vi "MEMR-Plot Gain Spectra.vi"(0 "Gain spectra in":cluster{"Freq (Hz)":dbl[], "Mag":dbl[][]}[](array[cluster]), 1 "Spectrum":refnum<vi>, 5 "Fmax":dbl=8000.0 format="%#_13g", 7 "Fpeak":dbl[](array[numeric]), 9 "Noise floor":cluster{"Freq (Hz)":dbl[], dbl[]}[](array[cluster]), 11 "error in (no error)":errorcluster, 12 "plotWhich":i32) -> (15 "error out":errorcluster)   [LabVIEW 2020]
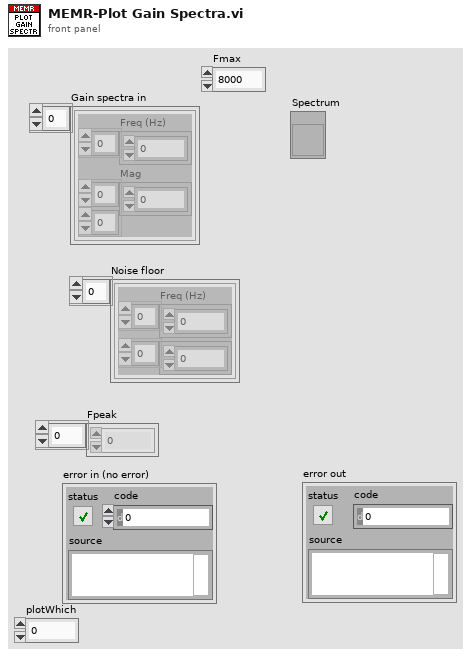
[diagram p1: front panel]
types:
  T1 = enum16{"User", "Prism", "Kelly", "Dark2", "Sequential", "Hue"}
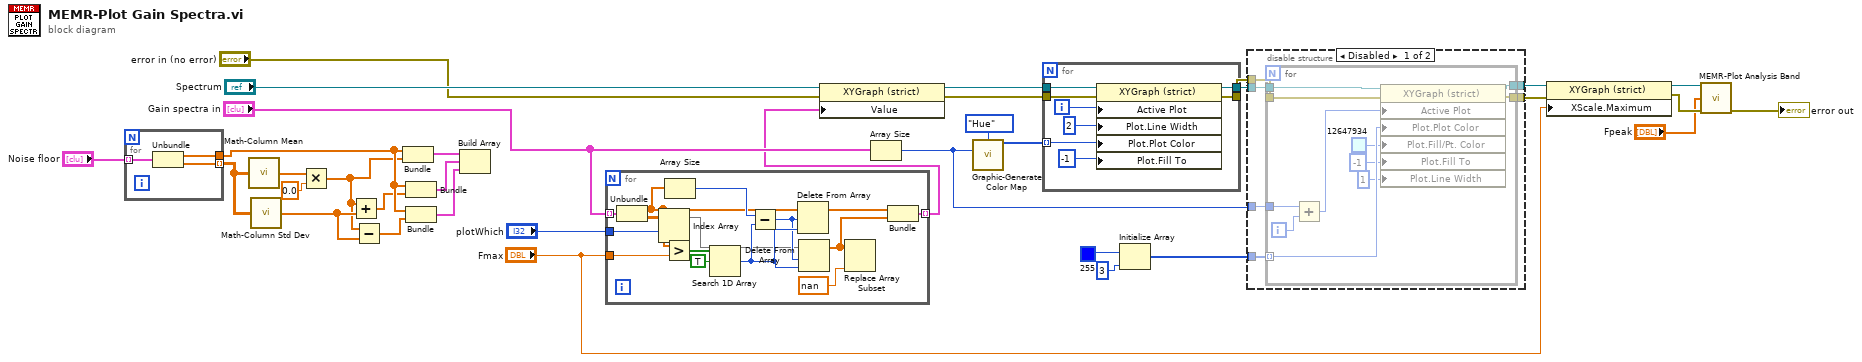
[diagram p0: block diagram]
diagram:
  n1 = for {
    tunnel: "Noise floor" -> [w37] mode=indexing
    tunnel: [w36] -> w23 mode=indexing
    tunnel: [w35] -> w24
    n2 = Unbundle(w37) -> ("Freq (Hz)"=w35:dbl[], w36:dbl[])
  }
  n3 = call "Math-Column Mean.vi"("2D Array"=w23) -> ("Column means"=w15:dbl[])
  n4 = call "Math-Column Std Dev.vi"("2D Array"=w23) -> ("Column means"=w16:dbl[])
  n5 = Multiply(x=w15, y=0.0) -> (x*y=w10:dbl[])
  n6 = Add(x=w10, y=w16) -> (x+y=w17:dbl[])
  n7 = Subtract(x=w10, y=w16) -> (x-y=w18:dbl[])
  n8 = Bundle("Freq (Hz)"=w24, w10) -> (w19:cluster{"Freq (Hz)":dbl[], dbl[]})  [unwired: 1 in]
  n9 = Bundle("Freq (Hz)"=w24, w17) -> (w20:cluster{"Freq (Hz)":dbl[], dbl[]})  [unwired: 1 in]
  n10 = Bundle("Freq (Hz)"=w24, w18) -> (w21:cluster{"Freq (Hz)":dbl[], dbl[]})  [unwired: 1 in]
  n11 = Build Array(w19, w20, w21) -> ()  [unwired: 1 out]
  n12 = for {
    tunnel: "Gain spectra in" -> [w52] mode=indexing
    tunnel: [w47] -> w1 mode=indexing
    tunnel: "Fmax" -> [w42]
    tunnel: "plotWhich" -> [w41]
    n13 = Unbundle(w52) -> ("Freq (Hz)"=w40:dbl[], "Mag"=w49:dbl[][])
    n14 = Index Array(array=w49, index (row)=w41) -> (element=w39:dbl[])  [unwired: 1 in]
    n15 = Greater?(x=w40, y=w42) -> (0:w51:bool[])
    n16 = Array Size(array=w40) -> (size(s)=w46:i32)
    n17 = Search 1D Array(1D array=w51, element=TRUE) -> (index of element=w45:i32)  [unwired: 1 in]
    n18 = Subtract(x=w46, y=w45) -> (x-y=w44:i32)
    n19 = Delete From Array(array=w40, length=w44, index=w45) -> (array with subset deleted=w48:dbl[])  [unwired: 1 out]
    n20 = Delete From Array(array=w39, length=w44, index=w45) -> (array with subset deleted=w38:dbl[])  [unwired: 1 out]
    n21 = Replace Array Subset(array=w38, new element=nan) -> ()  [unwired: 1 in, 1 out]
    n22 = Bundle("Freq (Hz)"=w48, "Mag"=w38) -> (w47:cluster{"Freq (Hz)":dbl[], "Mag":dbl[]})  [unwired: 1 in]
  }
  n23 = property on="Property Node" class="XYGraph (strict)"(reference="Spectrum", error in="error in (no error)", "Value"=w1) -> (reference out=w14:refnum<vi>, error out=w31:errorcluster)
  n24 = Array Size(array="Gain spectra in") -> (size(s)=w25:i32)
  n25 = call "Graphic-Generate Color Map.vi"("Map"=T1."Hue", "Size"=w25) -> ("Colors"=w32:u32[])  [unwired: 13 in]
  n26 = for {
    tunnel: w32 -> [w58] mode=indexing
    tunnel: w31 -> [w57]
    tunnel: [w56] -> w28
    tunnel: w14 -> [w54]
    tunnel: [w53] -> w13
    i -> [w60]
    n27 = property on="Property Node" class="XYGraph (strict)"(reference=w54, error in=w57, "Active Plot"=w60, "Plot.Line Width"=u8 2, "Plot.Plot Color"=w58, "Plot.Fill To"=i16 -1) -> (reference out=w53:refnum<vi>, error out=w56:errorcluster)
  }
  n28 = Initialize Array(u32 255, 3) -> (w27:u32[])
  n29 = disable-structure shown="Disabled" {
    disable-tunnel: w28 -> [w66 w78]
    disable-tunnel: w27 -> [w65 _]
    disable-tunnel: [w64 w78] -> w26
    disable-tunnel: w25 -> [w63 _]
    disable-tunnel: w13 -> [w62 w79]
    disable-tunnel: [w61 w79] -> w12
    frame Disabled {
      n30 = for {
        tunnel: w66 -> [w77]
        tunnel: w65 -> [w73] mode=indexing
        tunnel: w63 -> [w76]
        tunnel: [w69] -> w64
        tunnel: w62 -> [w68]
        tunnel: [w67] -> w61
        i -> [w75]
        n31 = Add(x=w76, y=w75) -> (x+y=w74:i32)
        n32 = property on="Property Node" class="XYGraph (strict)"(reference=w68, error in=w77, "Active Plot"=w74, "Plot.Plot Color"=w73, "Plot.Fill/Pt. Color"=u32 12647934, "Plot.Fill To"=i16 -1, "Plot.Line Width"=u8 1) -> (reference out=w67:refnum<vi>, error out=w69:errorcluster)
      }
    }
    frame Enabled {
    }
  }
  n33 = property on="Property Node" class="XYGraph (strict)"(reference=w12, error in=w26, "XScale.Maximum"="Fmax") -> (reference out=w6:refnum<vi>, error out=w5:errorcluster)
  n34 = call "MEMR-Plot Analysis Band.vi"("XYGraph in"=w6, "Fpeak"="Fpeak", "error in (no error)"=w5) -> ("error out"=→"error out":errorcluster)  [unwired: 12 in]
